vi "Remove Quotes if Existing.vi"(1 "String":string) -> (0 "String out":string)   [LabVIEW 2015, in "YAML Parser.lvlib"]
uses:
  YAML Parser.lvlib
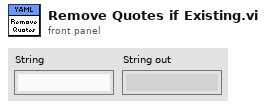
[diagram p1: front panel]
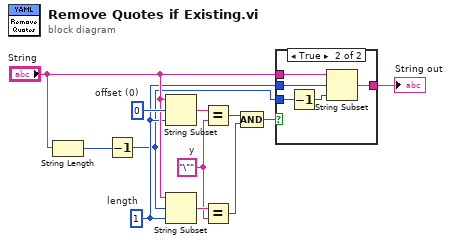
[diagram p0: block diagram]
diagram:
  w6 = "\""  # y
  w2 = 1  # length
  w12 = 0  # offset (0)
  n1 = String Length(string="String") -> (length=w11:i32)
  n2 = Decrement(x=w11) -> (x-1=w1:i32)
  n3 = String Subset(string="String", offset (0)=w12, length (rest)=w2) -> (substring=w9:string)
  n4 = String Subset(string="String", offset (0)=w1, length (rest)=w2) -> (substring=w10:string)
  n5 = Equal?(x=w9, y=w6) -> (x = y?=w8:bool)
  n6 = Equal?(x=w10, y=w6) -> (x = y?=w7:bool)
  n7 = Compound Arithmetic op=AND(w8, w7) -> (w5:bool)
  n8 = case shown="True" w5 {
    tunnel: [w13 w17] -> w4
    tunnel: "String" -> [w13 w18]
    tunnel: w2 -> [_ w16]
    tunnel: w1 -> [_ w15]
    frame False {
    }
    frame True {
      n9 = Decrement(x=w15) -> (x-1=w14:i32)
      n10 = String Subset(string=w18, offset (0)=w16, length (rest)=w14) -> (substring=w17:string)
    }
  }
  "String out" <- w4
